vi "Fin_OpenNRun.vi"(1 "VI name":string, 2 "ViDirPath":path) -> (0 "Execution:State":T1(ring))   [LabVIEW 2015]
panel:
  out "VI Path":path
  out "complete path":path
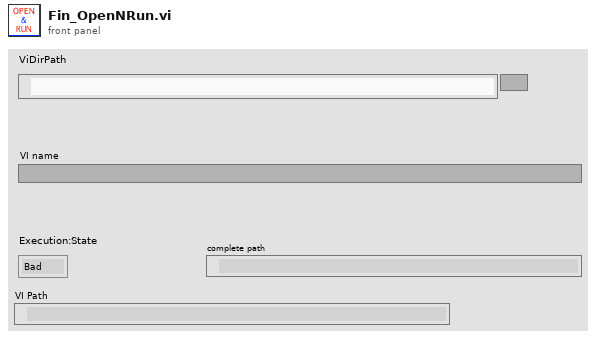
[diagram p1: front panel]
types:
  T1 = enum32{"Bad", "Idle", "Run top level", "Running"}
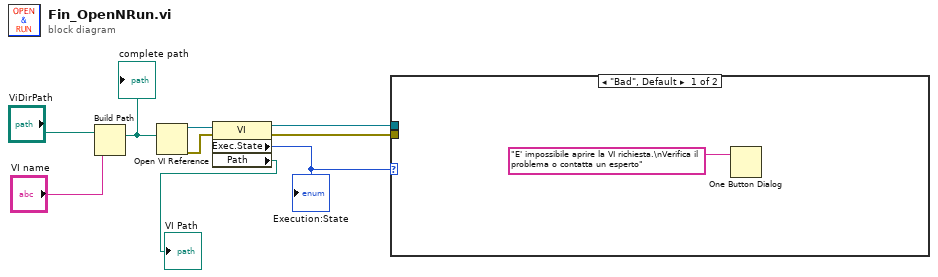
[diagram p0: block diagram]
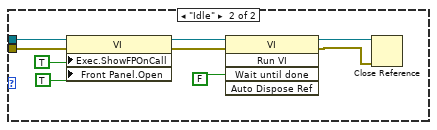
[diagram p2: hidden frame]
diagram:
  n1 = Build Path(base path="ViDirPath", name or relative path="VI name") -> (appended path=w6:path)
  "complete path" <- w6
  n2 = Open VI Reference(vi path=w6) -> (vi reference=w5:refnum<vi>, error out=w4:errorcluster)  [unwired: 5 in]
  n3 = property class="VI"(reference=w5, error in=w4) -> (reference out=w3:refnum<vi>, error out=w2:errorcluster, "Exec.State"=w7:T1, "Path"=→"VI Path":path)
  "Execution:State" <- w7
  n4 = case shown="\"Bad\", Default" w7 {
    tunnel: w3 -> [_ w15]
    tunnel: w2 -> [_ w14]
    frame "Bad", Default {
      n5 = One Button Dialog(message="E' impossibile aprire la VI richiesta.\nVerifica il problema o contatta un esperto") -> ()  [unwired: 1 in, 1 out]
    }
    frame "Idle" {
      n6 = property class="VI"(reference=w15, error in=w14, "Exec.ShowFPOnCall"=TRUE ("Execution:Show Front Panel On Load"), "Front Panel.Open"=TRUE ("Front Panel Window:Open")) -> (reference out=w16:refnum<vi>, error out=w13:errorcluster)
      n7 = invoke class="VI" method="Run VI"(reference=w16, error in=w13, "Wait until done"=FALSE ("Wait Until Done")) -> (reference out=w12:refnum<vi>, error out=w11:errorcluster)  [unwired: 2 in, 3 out]
      n8 = Close Reference(reference=w12, error in (no error)=w11) -> ()  [unwired: 1 out]
    }
  }
